vi "Set trigger.vi"(8 "error in (no error)":errorcluster, 11 "DAQOrcaFlash in":refnum<class "DAQOrcaFlash.lvclass">) -> (0 "error out":errorcluster, 3 "DAQOrcaFlash out":refnum<class "DAQOrcaFlash.lvclass">)   [LabVIEW 2012, in "DAQOrcaFlash.lvclass"]
uses:
  DAQOrcaFlash.lvclass
  DAQOrcaFlash.lvclass/DAQOrcaFlash.ctl
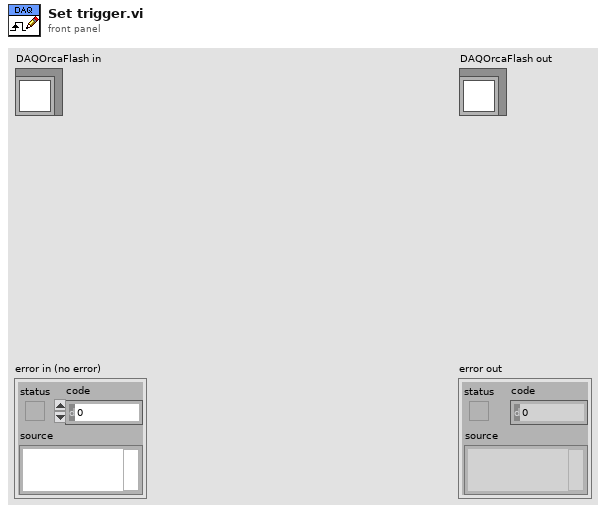
[diagram p1: front panel]
types:
  T1 = typedef "DAQOrcaFlash.lvclass/trigger_mode.ctl" = sgl
  T2 = typedef "DAQOrcaFlash.lvclass/trigger_source.ctl" = sgl
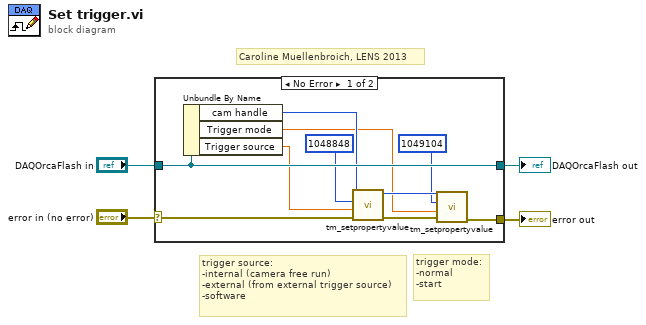
[diagram p0: block diagram]
diagram:
  # "trigger mode:\n-normal\n-start"
  # "trigger source:\n-internal (camera free run) \n-external (from external trigger source)\n-software"
  # "Caroline Muellenbroich, LENS 2013"
  n1 = case shown="No Error" "error in (no error)" {
    selector: "error in (no error)" -> [w9 w16]
    tunnel: [w7 w16] -> w3
    tunnel: [w14 w15] -> w1
    tunnel: "DAQOrcaFlash in" -> [w14 w15]
    frame No Error {
      n2 = Unbundle By Name(w14) -> ("cam handle"=w13:u32, "Trigger mode"=w5:T1, "Trigger source"=w6:T2)
      n3 = call <userlib>:"tm_setpropertyvalue.vi"("error in (no error)"=w9, "Value in"=w6, "Property ID"=u32 1048848, "Handle in"=w13) -> ("error out"=w8:errorcluster, "Handle out"=w12:u32)  [unwired: 6 in]
      n4 = call <userlib>:"tm_setpropertyvalue.vi"("error in (no error)"=w8, "Value in"=w5, "Property ID"=u32 1049104, "Handle in"=w12) -> ("error out"=w7:errorcluster)  [unwired: 6 in, 1 out]
    }
    frame Error {
    }
  }
  "error out" <- w3
  "DAQOrcaFlash out" <- w1
